vi "ToLog.vi"(10 "Amplituda":dbl, 11 "Pole vystupniho napeti":dbl[](array[numeric])) -> (3 "Napeti log":dbl[](array[numeric]))   [LabVIEW 2021]
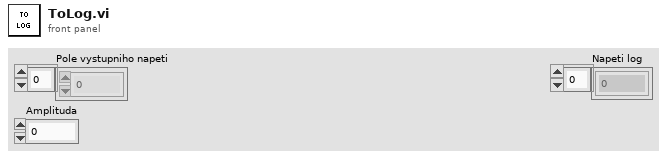
[diagram p1: front panel]
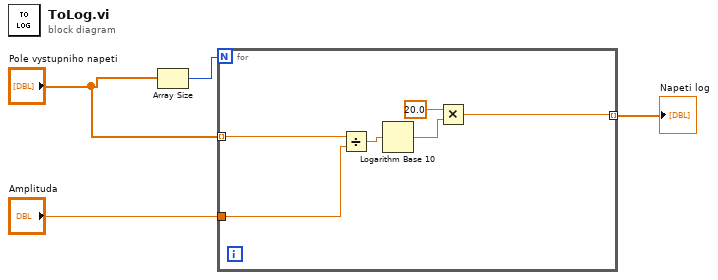
[diagram p0: block diagram]
diagram:
  n1 = Array Size(array="Pole vystupniho napeti") -> (size(s)=w3:i32)
  n2 = for {
    N: w3 -> [_]
    tunnel: "Pole vystupniho napeti" -> [w7] mode=indexing
    tunnel: "Amplituda" -> [w6]
    tunnel: [w5] -> w1 mode=indexing
    n3 = Divide(x=w7, y=w6) -> (x/y=w10:dbl)
    n4 = Logarithm Base 10(1:w10) -> (0:w9:dbl)
    n5 = Multiply(x=20.0, y=w9) -> (x*y=w5:dbl)
  }
  "Napeti log" <- w1
